vi "Collect coinc hunt results.vi"(11 "Dequeued elements":T1[](array[typedef])) -> (3 "Coincidences":T2[](array[typedef]))   [LabVIEW 2016]
uses:
  Typedefs/Coincidence.ctl
  Typedefs/Primary channel coincidence hunt.ctl
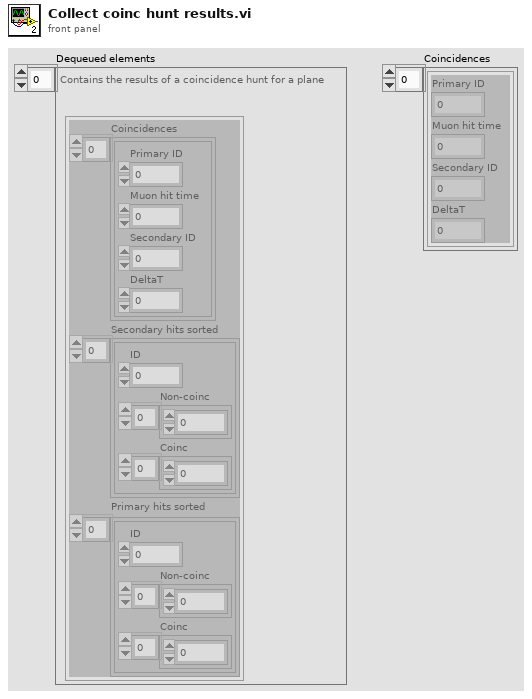
[diagram p1: front panel]
types:
  T1 = typedef "Primary channel coincidence hunt.ctl" = cluster{"Coincidences":T2[], "Secondary hits sorted":cluster{"ID":i8, "Non-coinc":u64[], "Coinc":u64[]}[], "Primary hits sorted":cluster{"ID":i8, "Non-coinc":u64[], "Coinc":u64[]}[]}
  T2 = typedef "Coincidence.ctl" = cluster{"Primary ID":i8, "Muon hit time":u64, "Secondary ID":i8, "DeltaT":i32}
  T3 = cluster{"ID":i8, "Non-coinc":i64[], "Coinc":i64[]}
  T4 = cluster{"ID":i8, "Non-coinc":u64[], "Coinc":u64[]}[]
  T5 = cluster{"ID":i8, "Non-coinc":u64[], "Coinc":u64[]}
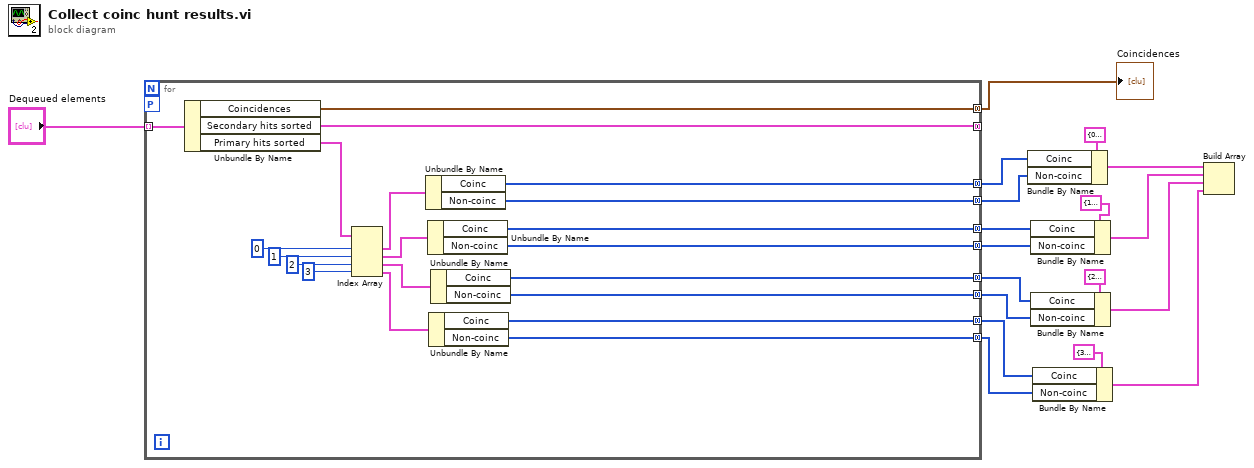
[diagram p0: block diagram]
diagram:
  n1 = for {
    tunnel: "Dequeued elements" -> [w38] mode=indexing
    tunnel: [w37] -> w18 mode=concatenating
    tunnel: [w36] -> _ mode=concatenating
    workers-P: _ -> [_]
    tunnel: [w29] -> w15 mode=concatenating
    tunnel: [w28] -> w14 mode=concatenating
    tunnel: [w26] -> w13 mode=concatenating
    tunnel: [w27] -> w12 mode=concatenating
    tunnel: [w25] -> w11 mode=concatenating
    tunnel: [w24] -> w10 mode=concatenating
    tunnel: [w22] -> w9 mode=concatenating
    tunnel: [w23] -> w8 mode=concatenating
    n2 = Unbundle By Name(w38) -> ("Coincidences"=w37:T2[], "Secondary hits sorted"=w36:T4, "Primary hits sorted"=w35:T4)
    n3 = Index Array(array=w35, index #1=0 ("index"), index #2=1 ("index"), index #3=2 ("index"), index #4=3 ("index")) -> (element #1=w30:T5, element #2=w21:T5, element #3=w20:T5, element #4=w19:T5)
    n4 = Unbundle By Name(w30) -> ("Coinc"=w29:u64[], "Non-coinc"=w28:u64[])
    n5 = Unbundle By Name(w21) -> ("Coinc"=w26:u64[], "Non-coinc"=w27:u64[])
    n6 = Unbundle By Name(w19) -> ("Coinc"=w22:u64[], "Non-coinc"=w23:u64[])
    n7 = Unbundle By Name(w20) -> ("Coinc"=w25:u64[], "Non-coinc"=w24:u64[])
  }
  "Coincidences" <- w18
  n8 = Bundle By Name(cluster=T3 {"ID"=0, "Non-coinc"=[], "Coinc"=[]} ("element"), "Coinc"=w15, "Non-coinc"=w14) -> (w4:T3)
  n9 = Bundle By Name(cluster=T3 {"ID"=1, "Non-coinc"=[], "Coinc"=[]} ("element"), "Coinc"=w13, "Non-coinc"=w12) -> (w3:T3)
  n10 = Bundle By Name(cluster=T3 {"ID"=2, "Non-coinc"=[], "Coinc"=[]} ("element"), "Coinc"=w11, "Non-coinc"=w10) -> (w2:T3)
  n11 = Bundle By Name(cluster=T3 {"ID"=3, "Non-coinc"=[], "Coinc"=[]} ("element"), "Coinc"=w9, "Non-coinc"=w8) -> (w1:T3)
  n12 = Build Array(w4, w3, w2, w1) -> ()  [unwired: 1 out]
